vi "AVQ8347 Average On Off.vi"(8 "Error In":errorcluster, 10 "Processing Select (OFF)":bool, 11 "VISA Session":refnum<visa-resource-name>) -> (0 "Error Out":errorcluster, 2 "Send Code":string, 3 "Copy VISA Session":refnum<visa-resource-name>)   [LabVIEW 2018]
doc: "Average processing Implementation start Implementation stop"
panel:
  # "Averege On Off"
  # "ON\nOFF"
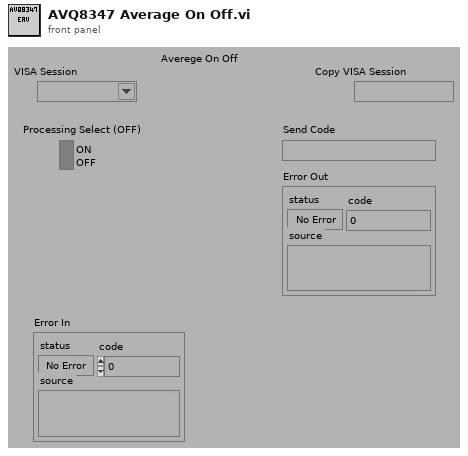
[diagram p1: front panel]
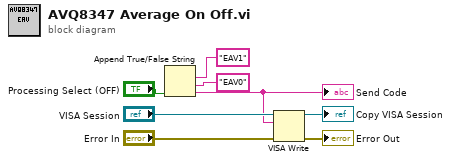
[diagram p0: block diagram]
diagram:
  n1 = Append True/False String(1:"Processing Select (OFF)", 2:"EAV0", 3:"EAV1") -> (0:w1:string)  [unwired: 1 in]
  "Send Code" <- w1
  n2 = VISA Write(VISA resource name="VISA Session", write buffer=w1, error in (no error)="Error In") -> (VISA resource name out=→"Copy VISA Session":refnum<visa-resource-name>, error out=→"Error Out":errorcluster)  [unwired: 1 out]
